vi "Pump Fast Forward.vi"(4 "Time Target (s)":dbl=10.0 format="%#_13g", 5 "Init":bool, 6 "percent":dbl=1.0 format="%#_13g", 7 "Direction":T1, 8 "error in (no error)":errorcluster, 9 "Leak":bool, 11 "Stand in":refnum<class "Stand.lvclass">) -> (0 "error out":errorcluster, 2 "Done":bool caption="Time has Elapsed")   [LabVIEW 2019, in "Stand.lvclass"]
uses:
  Stand.lvclass
  C:/Users/ANENKOV_V1/Desktop/src/Device_class/Device.lvclass
  TypeDef/Direction.ctl
  Device_class/Device.lvclass/Device.ctl
  Stand.lvclass/Stand.ctl
  AI_class/AI.lvclass/AI.ctl
  AnalogComparator_class/AnalogComparator.lvclass/AnalogComparator.ctl
  FPGA/TypeDef/AI index.ctl
  AnalogComparator_class/GetStatus.vi
  FPGA_API_class/FPGA API.lvclass
  Device_class/Device.lvclass
  AI_class/AI.lvclass
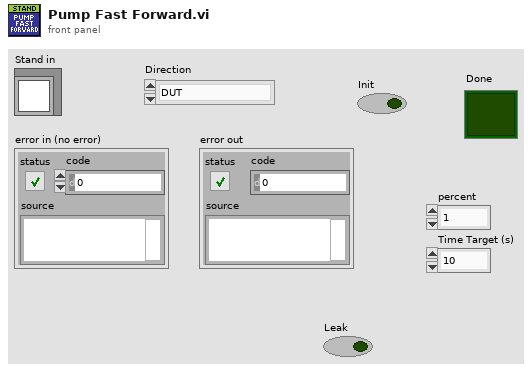
[diagram p1: front panel]
types:
  T1 = typedef "Direction.ctl" = enum8{"DUT", "Chamber"}
  T2 = typedef "AI_Data.ctl" = cluster{"Stat Data":T3, "OutOfRangeMax":bool, "OutOfRangeMin":bool, "HIHI":bool, "HI":bool, "LO":bool, "LOLO":bool}
  T3 = typedef "AI Statistics Data.ctl" = cluster{"raw mean":dbl, "scl mean":dbl, "raw mean 1Hz":dbl, "scl mean 1Hz":dbl}
  T4 = typedef "AI index.ctl" = u8
  T5 = typedef "Setting Pressure PI.ctl" = cluster{"A [MPa/V]":dbl, "P0 [MPa]":dbl}
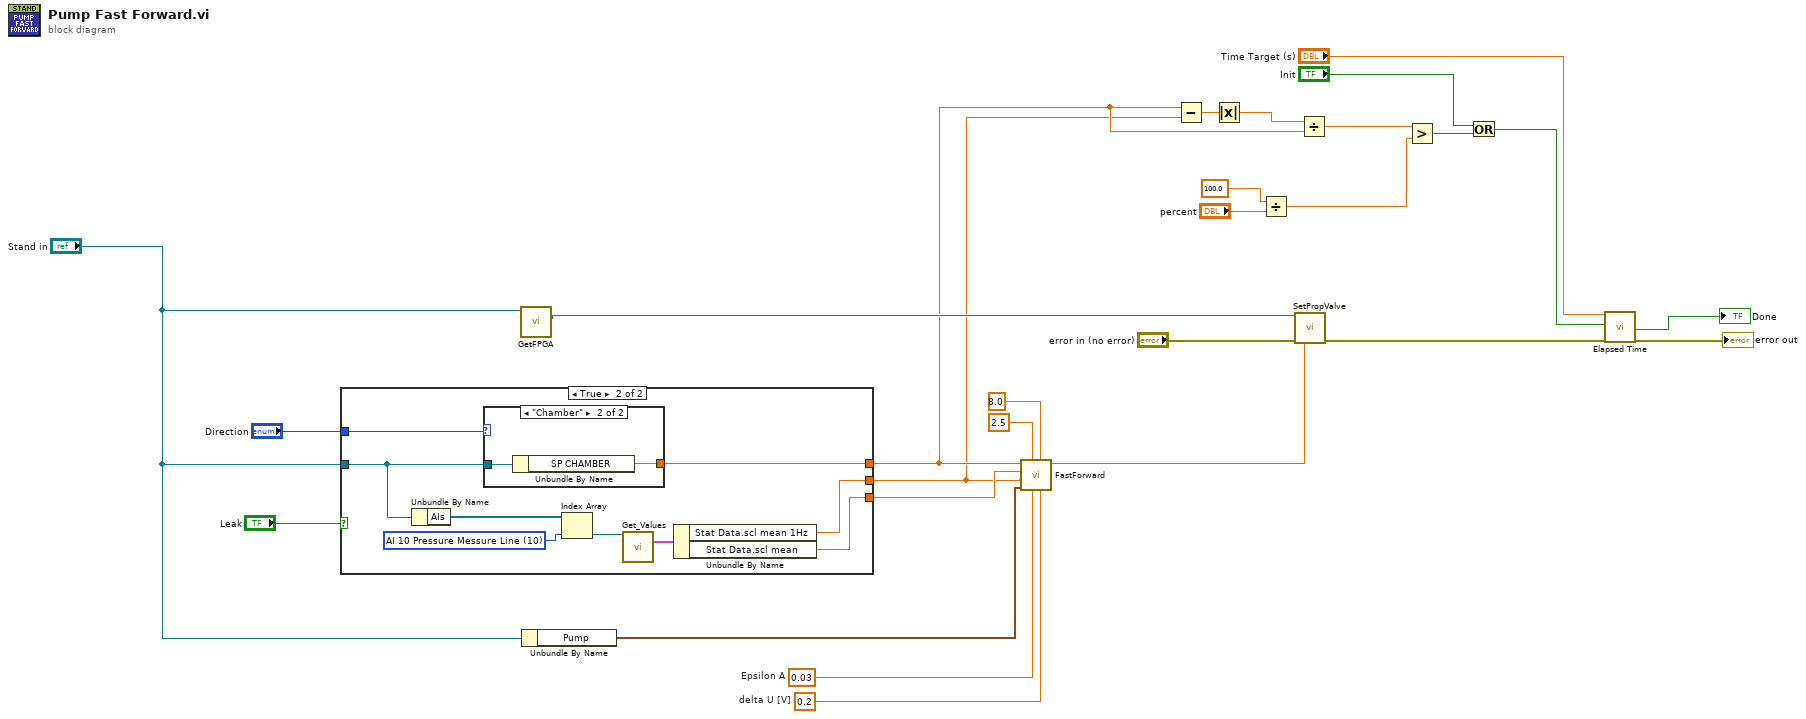
[diagram p0: block diagram]
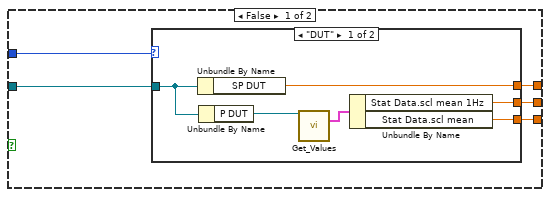
[diagram p2: hidden frame]
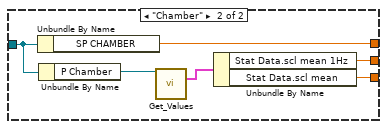
[diagram p3: hidden frame]
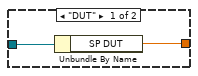
[diagram p4: hidden frame]
diagram:
  w26 = 0.2  # delta U [V]
  w25 = 0.03  # Epsilon A
  n1 = case shown="True" "Leak" {
    tunnel: "Stand in" -> [w32 w48]
    tunnel: "Direction" -> [w31 w53]
    tunnel: [w30 w52] -> w9
    tunnel: [w29 w49] -> w8
    tunnel: [w28 w50] -> w1
    frame False {
      n2 = case shown="\"DUT\"" w31 {
        tunnel: [w38 w44] -> w29
        tunnel: [w36 w42] -> w30
        tunnel: w32 -> [w35 w41]
        tunnel: [w33 w39] -> w28
        frame "DUT" {
          n3 = Unbundle By Name(w35) -> ("SP DUT"=w36:dbl)
          n4 = Unbundle By Name(w35) -> ("P DUT"=w34:refnum<class "AI.lvclass">)
          n5 = call "Get_Values.vi"("reference in"=w34) -> ("Data"=w37:T2)  [unwired: 14 in]
          n6 = Unbundle By Name(w37) -> ("Stat Data.scl mean 1Hz"=w33:dbl, "Stat Data.scl mean"=w38:dbl)
        }
        frame "Chamber" {
          n7 = Unbundle By Name(w41) -> ("SP CHAMBER"=w42:dbl)
          n8 = Unbundle By Name(w41) -> ("P Chamber"=w40:refnum<class "AI.lvclass">)
          n9 = call "Get_Values.vi"("reference in"=w40) -> ("Data"=w43:T2)  [unwired: 14 in]
          n10 = Unbundle By Name(w43) -> ("Stat Data.scl mean 1Hz"=w39:dbl, "Stat Data.scl mean"=w44:dbl)
        }
      }
    }
    frame True {
      w46 = T4 10 items=["AI 0 Cooling Station Level", "AI 1 Cooling Station Temp", "AI 2 Oil Supply Level", "AI 3 Oil Supply Temp", "AI 4 ", "AI 5 Pressure Haskel", "AI 6 Pressure DUT", "AI 7 Pressure Chamber", "AI 8 Pressure Air inlet", "AI 9 Pressure Air outlet", "AI 10 Pressure Messure Line", "AI 11 DUT 2", "AI 12 Chamber 2"] ("AI index")
      n11 = Unbundle By Name(w48) -> ("AIs"=w47:refnum<class "AI.lvclass">[])
      n12 = case shown="\"Chamber\"" w53 {
        tunnel: [w55 w57] -> w52
        tunnel: w48 -> [w54 w56]
        frame "DUT" {
          n13 = Unbundle By Name(w54) -> ("SP DUT"=w55:dbl)
        }
        frame "Chamber" {
          n14 = Unbundle By Name(w56) -> ("SP CHAMBER"=w57:dbl)
        }
      }
      n15 = Index Array(array=w47, index=w46) -> (element=w45:refnum<class "AI.lvclass">)
      n16 = call "Get_Values.vi"("reference in"=w45) -> ("Data"=w51:T2)  [unwired: 14 in]
      n17 = Unbundle By Name(w51) -> ("Stat Data.scl mean 1Hz"=w50:dbl, "Stat Data.scl mean"=w49:dbl)
    }
  }
  n18 = call "GetFPGA.vi"("Device in"="Stand in") -> ("FPGA API.lvclass"=w22:refnum<class "FPGA API.lvclass">)  [unwired: 10 in]
  n19 = Unbundle By Name("Stand in") -> ("Pump"=w21:T5)
  n20 = call "FastForward.vi"("delta U [V]"=w26, "U max [V]"=8.0, "Epsilon A"=w25, "U min [V]"=2.5, "Setting"=w21, "Mean"=w1, "PV"=w8, "SP"=w9) -> ("U"=w23:dbl)  [unwired: 3 in]
  n21 = Subtract(x=w9, y=w1) -> (x-y=w18:dbl)
  n22 = Absolute Value(x=w18) -> (abs(x)=w17:dbl)
  n23 = Divide(x=100.0, y="percent") -> (x/y=w5:dbl)
  n24 = call-dynamic "SetPropValve.vi"("FPGA API in"=w22, "error in (no error)"="error in (no error)", "AO 1"=w23) -> ("error out"=w7:errorcluster)  [unwired: 11 in, 1 out]
  n25 = Divide(x=w17, y=w9) -> (x/y=w16:dbl)
  n26 = Greater?(x=w16, y=w5) -> (0:w14:bool)
  n27 = Or(x="Init", y=w14) -> (x .or. y?=w13:bool)
  n28 = call "Elapsed Time"("Time Target (s)"="Time Target (s)", "Reset"=w13, "error in (no error)"=w7) -> ("Time has Elapsed"=→"Done":bool, "error out"=→"error out":errorcluster)  [unwired: 9 in, 6 out]
